vi "Number_calc.vi"() -> ()   [LabVIEW 2016]
panel:
  in  "file path (use dialog) 3":path
  in  "file path (use dialog) 2":path
  in  "ON/OFF":bool
  out "?":bool
  in  "CLEAR":bool
  out "ans":dbl
  out "Y":dbl
  in  "?":bool
  out "X":dbl
  out "ope":string
  in  "?":bool
  in  "?":bool
  in  "?":bool
  in  "?":bool
  out "INPUT(X & Y)":string
  in  "?":bool
  in  "?":bool
  in  "?":bool
  in  "?":bool
  in  "?":bool
  in  "?":bool
  in  "?":bool
  in  "?":bool
  in  "?":bool
  in  "?":bool
  in  "file path (use dialog)":path
  # "CALCULATOR"
  # "Please Ensure The \nBUTTON is ON"
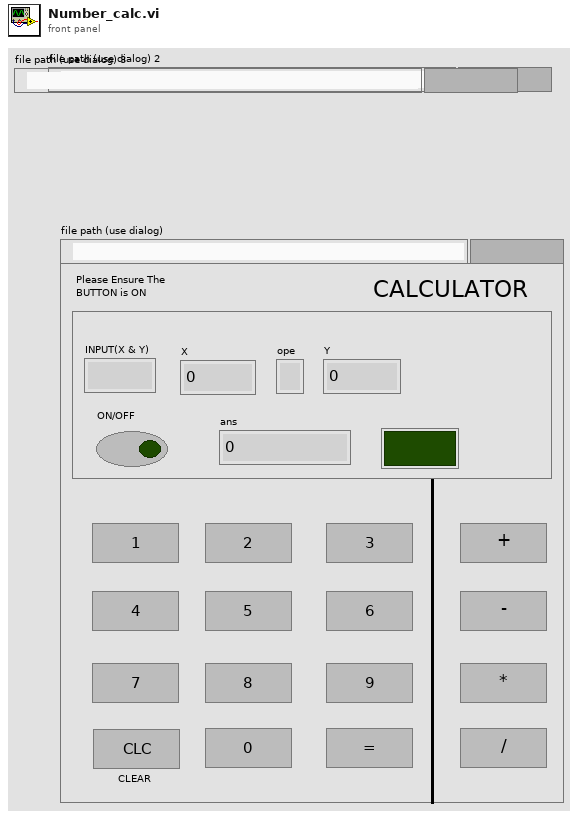
[diagram p1: front panel]
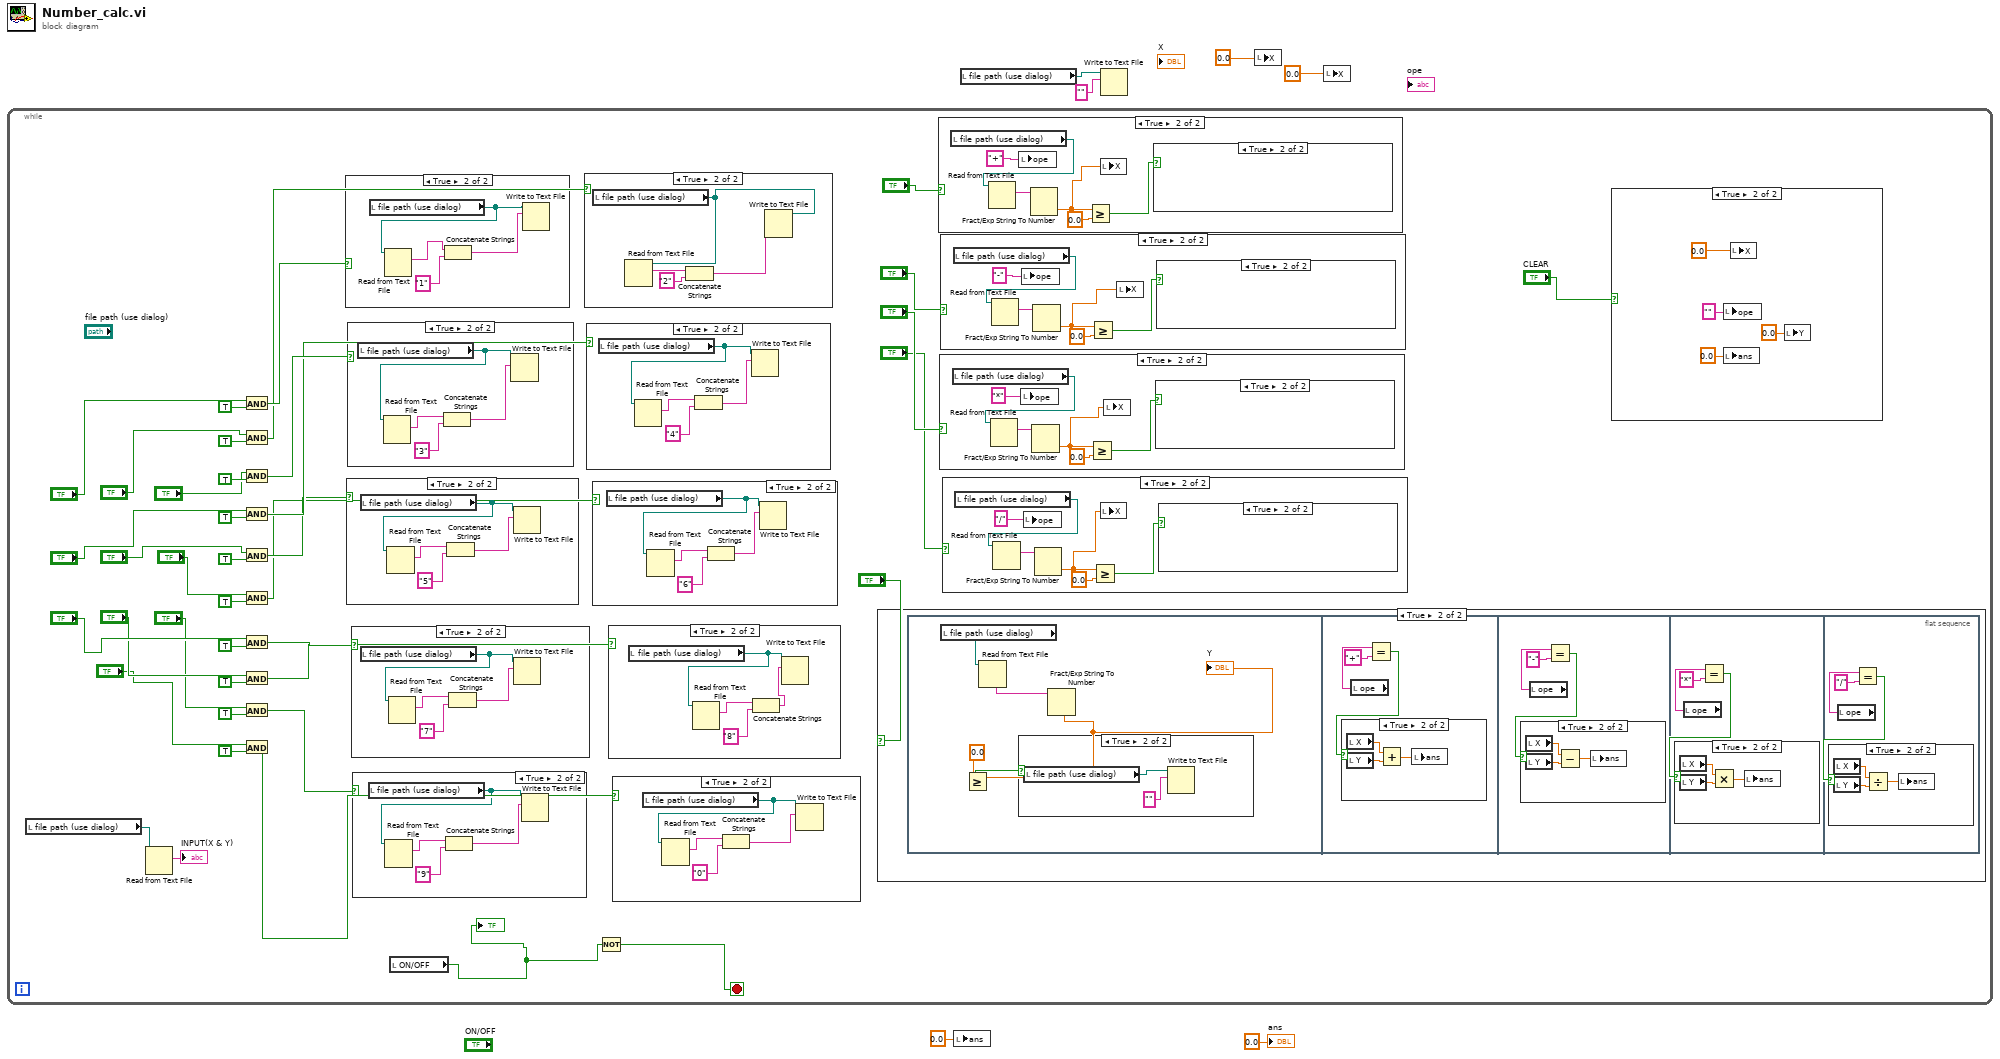
[diagram p0: block diagram]
diagram:
  n1 = while {
    stop <- w8 stop-if-true
    n2 = local read "file path (use dialog)"() -> (w16:path)
    n3 = Read from Text File(file (use dialog)=w16) -> (text=→"INPUT(X & Y)":string)  [unwired: 3 in, 3 out]
    n4 = And(x="?", y=TRUE) -> (x .and. y?=w26:bool)
    n5 = And(x="?", y=TRUE) -> (x .and. y?=w25:bool)
    n6 = And(x="?", y=TRUE) -> (x .and. y?=w24:bool)
    n7 = And(x="?", y=TRUE) -> (x .and. y?=w23:bool)
    n8 = And(x="?", y=TRUE) -> (x .and. y?=w22:bool)
    n9 = And(x="?", y=TRUE) -> (x .and. y?=w21:bool)
    n10 = And(x="?", y=TRUE) -> (x .and. y?=w20:bool)
    n11 = And(x="?", y=TRUE) -> (x .and. y?=w19:bool)
    n12 = And(x="?", y=TRUE) -> (x .and. y?=w18:bool)
    n13 = And(x="?", y=TRUE) -> (x .and. y?=w17:bool)
    n14 = case shown="True" w26 {
      frame False {
      }
      frame True {
        n15 = local read "file path (use dialog)"() -> (w149:path)
        n16 = Read from Text File(file (use dialog)=w149) -> (text=w148:string)  [unwired: 3 in, 3 out]
        n17 = Concatenate Strings(w148, "1" ("text")) -> (w146:string)
        n18 = Write to Text File(file (use dialog)=w149, text=w146) -> ()  [unwired: 2 in, 3 out]
      }
    }
    n19 = case shown="True" w22 {
      frame False {
      }
      frame True {
        n20 = local read "file path (use dialog)"() -> (w130:path)
        n21 = Read from Text File(file (use dialog)=w130) -> (text=w133:string)  [unwired: 3 in, 3 out]
        n22 = Concatenate Strings(w133, "5" ("text")) -> (w131:string)
        n23 = Write to Text File(file (use dialog)=w130, text=w131) -> ()  [unwired: 2 in, 3 out]
      }
    }
    n24 = case shown="True" w24 {
      frame False {
      }
      frame True {
        n25 = local read "file path (use dialog)"() -> (w139:path)
        n26 = Read from Text File(file (use dialog)=w139) -> (text=w138:string)  [unwired: 3 in, 3 out]
        n27 = Concatenate Strings(w138, "3" ("text")) -> (w140:string)
        n28 = Write to Text File(file (use dialog)=w139, text=w140) -> ()  [unwired: 2 in, 3 out]
      }
    }
    n29 = case shown="True" w20 {
      frame False {
      }
      frame True {
        n30 = local read "file path (use dialog)"() -> (w122:path)
        n31 = Read from Text File(file (use dialog)=w122) -> (text=w125:string)  [unwired: 3 in, 3 out]
        n32 = Concatenate Strings(w125, "7" ("text")) -> (w123:string)
        n33 = Write to Text File(file (use dialog)=w122, text=w123) -> ()  [unwired: 2 in, 3 out]
      }
    }
    n34 = case shown="True" w18 {
      frame False {
      }
      frame True {
        n35 = local read "file path (use dialog)"() -> (w115:path)
        n36 = Read from Text File(file (use dialog)=w115) -> (text=w117:string)  [unwired: 3 in, 3 out]
        n37 = Concatenate Strings(w117, "9" ("text")) -> (w114:string)
        n38 = Write to Text File(file (use dialog)=w115, text=w114) -> ()  [unwired: 2 in, 3 out]
      }
    }
    n39 = local read "ON/OFF"() -> (w7:bool)
    "?" <- w7
    n40 = case shown="True" w25 {
      frame False {
      }
      frame True {
        n41 = local read "file path (use dialog)"() -> (w142:path)
        n42 = Read from Text File(file (use dialog)=w142) -> (text=w144:string)  [unwired: 3 in, 3 out]
        n43 = Concatenate Strings(w144, "2" ("text")) -> (w143:string)
        n44 = Write to Text File(file (use dialog)=w142, text=w143) -> ()  [unwired: 2 in, 3 out]
      }
    }
    n45 = case shown="True" w23 {
      frame False {
      }
      frame True {
        n46 = local read "file path (use dialog)"() -> (w135:path)
        n47 = Read from Text File(file (use dialog)=w135) -> (text=w137:string)  [unwired: 3 in, 3 out]
        n48 = Concatenate Strings(w137, "4" ("text")) -> (w136:string)
        n49 = Write to Text File(file (use dialog)=w135, text=w136) -> ()  [unwired: 2 in, 3 out]
      }
    }
    n50 = case shown="True" w21 {
      frame False {
      }
      frame True {
        n51 = local read "file path (use dialog)"() -> (w126:path)
        n52 = Read from Text File(file (use dialog)=w126) -> (text=w128:string)  [unwired: 3 in, 3 out]
        n53 = Concatenate Strings(w128, "6" ("text")) -> (w127:string)
        n54 = Write to Text File(file (use dialog)=w126, text=w127) -> ()  [unwired: 2 in, 3 out]
      }
    }
    n55 = Not(x=w7) -> (.not. x?=w8:bool)
    n56 = case shown="True" w19 {
      frame False {
      }
      frame True {
        n57 = local read "file path (use dialog)"() -> (w118:path)
        n58 = Read from Text File(file (use dialog)=w118) -> (text=w120:string)  [unwired: 3 in, 3 out]
        n59 = Concatenate Strings(w120, "8" ("text")) -> (w119:string)
        n60 = Write to Text File(file (use dialog)=w118, text=w119) -> ()  [unwired: 2 in, 3 out]
      }
    }
    n61 = case shown="True" w17 {
      frame False {
      }
      frame True {
        n62 = local read "file path (use dialog)"() -> (w110:path)
        n63 = Read from Text File(file (use dialog)=w110) -> (text=w112:string)  [unwired: 3 in, 3 out]
        n64 = Concatenate Strings(w112, "0" ("text")) -> (w111:string)
        n65 = Write to Text File(file (use dialog)=w110, text=w111) -> ()  [unwired: 2 in, 3 out]
      }
    }
    n66 = case shown="True" "?" {
      frame False {
      }
      frame True {
        n67 = flat-sequence {
          frame #0 {
            n68 = local read "file path (use dialog)"() -> (w73:path)
            n69 = Read from Text File(file (use dialog)=w73) -> (text=w74:string)  [unwired: 3 in, 3 out]
            n70 = Fract/Exp String To Number(string=w74) -> (number=w77:dbl)  [unwired: 3 in, 1 out]
            "Y" <- w77
            n71 = Greater Or Equal?(x=w77, y=0.0) -> (x >= y?=w76:bool)
            n72 = case shown="True" w76 {
              frame False {
              }
              frame True {
                n73 = local read "file path (use dialog)"() -> (w78:path)
                n74 = Write to Text File(file (use dialog)=w78, text="") -> ()  [unwired: 2 in, 3 out]
              }
            }
          }
          frame #1 {
            n75 = local read "ope"() -> (w82:string)
            n76 = Equal?(x=w82, y="+") -> (x = y?=w80:bool)
            n77 = case shown="True" w80 {
              frame False {
              }
              frame True {
                n78 = local read "X"() -> (w84:dbl)
                n79 = local read "Y"() -> (w85:dbl)
                n80 = Add(x=w84, y=w85) -> (x+y=w83:dbl)
                n81 = local write "ans"(w83) -> ()
              }
            }
          }
          frame #2 {
            n82 = local read "ope"() -> (w86:string)
            n83 = Equal?(x=w86, y="-") -> (x = y?=w88:bool)
            n84 = case shown="True" w88 {
              frame False {
              }
              frame True {
                n85 = local read "X"() -> (w90:dbl)
                n86 = local read "Y"() -> (w91:dbl)
                n87 = Subtract(x=w90, y=w91) -> (x-y=w89:dbl)
                n88 = local write "ans"(w89) -> ()
              }
            }
          }
          frame #3 {
            n89 = local read "ope"() -> (w94:string)
            n90 = Equal?(x=w94, y="*") -> (x = y?=w92:bool)
            n91 = case shown="True" w92 {
              frame False {
              }
              frame True {
                n92 = local read "X"() -> (w96:dbl)
                n93 = local read "Y"() -> (w97:dbl)
                n94 = Multiply(x=w96, y=w97) -> (x*y=w95:dbl)
                n95 = local write "ans"(w95) -> ()
              }
            }
          }
          frame #4 {
            n96 = local read "ope"() -> (w98:string)
            n97 = Equal?(x=w98, y="/") -> (x = y?=w100:bool)
            n98 = case shown="True" w100 {
              frame False {
              }
              frame True {
                n99 = local read "X"() -> (w102:dbl)
                n100 = local read "Y"() -> (w103:dbl)
                n101 = Divide(x=w102, y=w103) -> (x/y=w101:dbl)
                n102 = local write "ans"(w101) -> ()
              }
            }
          }
        }
      }
    }
    n103 = case shown="True" "?" {
      frame False {
      }
      frame True {
        n104 = local read "file path (use dialog)"() -> (w109:path)
        n105 = Read from Text File(file (use dialog)=w109) -> (text=w108:string)  [unwired: 3 in, 3 out]
        n106 = local write "ope"("+" ("text 2")) -> ()
        n107 = Fract/Exp String To Number(string=w108) -> (number=w104:dbl)  [unwired: 3 in, 1 out]
        n108 = Greater Or Equal?(x=w104, y=0.0) -> (x >= y?=w106:bool)
        n109 = local write "X"(w104) -> ()
        n110 = case shown="True" w106 {
          frame False {
          }
          frame True {
          }
        }
      }
    }
    n111 = case shown="True" "?" {
      frame False {
      }
      frame True {
        n112 = local read "file path (use dialog)"() -> (w66:path)
        n113 = Read from Text File(file (use dialog)=w66) -> (text=w65:string)  [unwired: 3 in, 3 out]
        n114 = local write "ope"("*" ("text 2")) -> ()
        n115 = Fract/Exp String To Number(string=w65) -> (number=w61:dbl)  [unwired: 3 in, 1 out]
        n116 = Greater Or Equal?(x=w61, y=0.0) -> (x >= y?=w63:bool)
        n117 = local write "X"(w61) -> ()
        n118 = case shown="True" w63 {
          frame False {
          }
          frame True {
          }
        }
      }
    }
    n119 = case shown="True" "?" {
      frame False {
      }
      frame True {
        n120 = local read "file path (use dialog)"() -> (w72:path)
        n121 = Read from Text File(file (use dialog)=w72) -> (text=w71:string)  [unwired: 3 in, 3 out]
        n122 = local write "ope"("-" ("text 2")) -> ()
        n123 = Fract/Exp String To Number(string=w71) -> (number=w67:dbl)  [unwired: 3 in, 1 out]
        n124 = Greater Or Equal?(x=w67, y=0.0) -> (x >= y?=w69:bool)
        n125 = local write "X"(w67) -> ()
        n126 = case shown="True" w69 {
          frame False {
          }
          frame True {
          }
        }
      }
    }
    n127 = case shown="True" "?" {
      frame False {
      }
      frame True {
        n128 = local read "file path (use dialog)"() -> (w56:path)
        n129 = Read from Text File(file (use dialog)=w56) -> (text=w55:string)  [unwired: 3 in, 3 out]
        n130 = local write "ope"("/" ("text 2")) -> ()
        n131 = Fract/Exp String To Number(string=w55) -> (number=w51:dbl)  [unwired: 3 in, 1 out]
        n132 = Greater Or Equal?(x=w51, y=0.0) -> (x >= y?=w53:bool)
        n133 = local write "X"(w51) -> ()
        n134 = case shown="True" w53 {
          frame False {
          }
          frame True {
            n135 = local read "file path (use dialog) 3"() -> (w57:path)
            n136 = local read "file path (use dialog) 2"() -> (w59:path)
            n137 = Write to Text File(file (use dialog)=w57, text="") -> ()  [unwired: 2 in, 3 out]
            n138 = Write to Text File(file (use dialog)=w59, text="") -> ()  [unwired: 2 in, 3 out]
          }
        }
      }
    }
    n139 = case shown="True" "CLEAR" {
      frame False {
      }
      frame True {
        n140 = local write "ope"("" ("ope")) -> ()
        n141 = local write "ans"(0.0 ("ans")) -> ()
        n142 = local write "X"(0.0 ("number")) -> ()
        n143 = local write "Y"(0.0 ("Y")) -> ()
      }
    }
  }
  n144 = local write "ans"(0.0 ("x+y")) -> ()
  n145 = local read "file path (use dialog)"() -> (w5:path)
  n146 = Write to Text File(file (use dialog)=w5, text="") -> ()  [unwired: 2 in, 3 out]
  n147 = local write "X"(0.0 ("number")) -> ()
  n148 = local write "X"(0.0 ("number")) -> ()
  "ans" <- 0.0 ("x+y")
